vi "Update Plot.vi"(8 "error in (no error)":errorcluster, 11 "Lockin Processor in":refnum<class "Lockin Processor.lvclass">) -> (0 "error out":errorcluster, 3 "Lockin Processor out":refnum<class "Lockin Processor.lvclass">)   [LabVIEW 2015, in "Lockin Processor.lvclass"]
uses:
  Lockin Processor.lvclass
  Lockin Processor.lvclass/Lockin Processor.ctl
  Lockin Processor Configuration.ctl
  Read Lockin Processor Configuration.vi
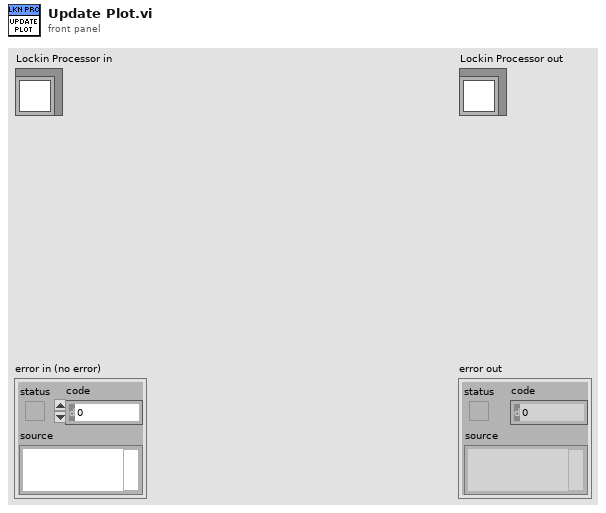
[diagram p1: front panel]
types:
  T1 = typedef "Lockin Processor Configuration.ctl" = cluster{"Time constant":dbl, "Phase":dbl, "Signal channels":string[], "Group":string, "X channel":string, "Live update":bool}
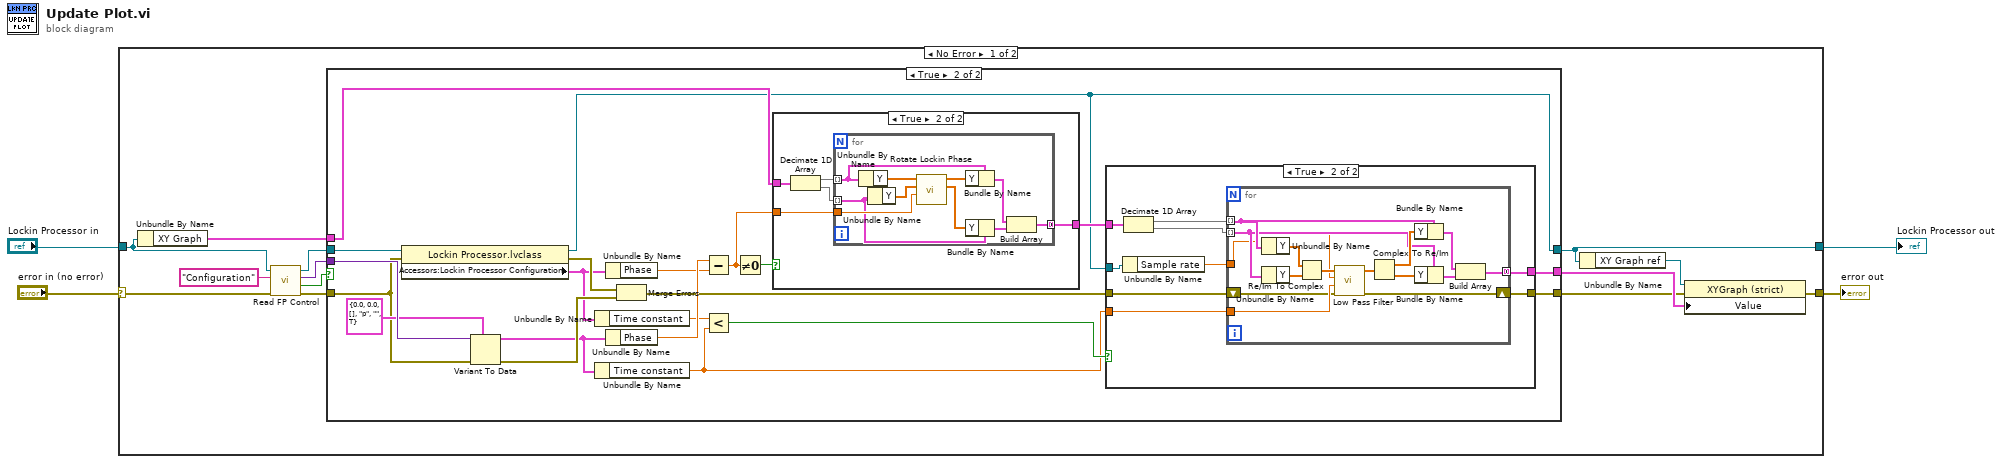
[diagram p0: block diagram]
diagram:
  n1 = case shown="No Error" "error in (no error)" {
    selector: "error in (no error)" -> [w7 w85]
    tunnel: [w6 w85] -> w3
    tunnel: [w9 w84] -> w1
    tunnel: "Lockin Processor in" -> [w10 w84]
    frame No Error {
      n2 = Unbundle By Name(w10) -> ("XY Graph"=w12:cluster{"X":dbl[], "Y":dbl[]}[])
      n3 = call-dynamic "Read FP Control.vi"("error in (no error)"=w7, "Control Name"="Configuration", "Measure Object in"=w10) -> ("error out"=w15:errorcluster, "Present"=w14:bool, "Control Value"=w16:variant, "Measure Object out"=w13:refnum<class "Lockin Processor.lvclass">)  [unwired: 5 in]
      n4 = case shown="True" w14 {
        tunnel: w16 -> [_ w41]
        tunnel: w15 -> [w18 w38]
        tunnel: w13 -> [w19 w39]
        tunnel: w12 -> [w20 w34]
        tunnel: [w19 w21] -> w9
        tunnel: [w20 w22] -> w11
        tunnel: [w18 w23] -> w5
        frame False {
        }
        frame True {
          n5 = property class="Lockin Processor.lvclass"(reference=w39, error in=w38) -> (reference out=w21:refnum<class "Lockin Processor.lvclass">, error out=w37:errorcluster, "Accessors:Lockin Processor Configuration"=w30:T1)
          n6 = Variant To Data(error in=w38, type=T1 {"Time constant"=0.0, "Phase"=0.0, "Signal channels"=[], "Group"="p", "X channel"="", "Live update"=TRUE} ("Configuration"), Variant=w41) -> (data=w29:T1, error out=w36:errorcluster)
          n7 = Unbundle By Name(w30) -> ("Time constant"=w28:dbl)
          n8 = Unbundle By Name(w29) -> ("Time constant"=w26:dbl)
          n9 = Unbundle By Name(w30) -> ("Phase"=w31:dbl)
          n10 = Unbundle By Name(w29) -> ("Phase"=w32:dbl)
          n11 = Merge Errors(w37, w36) -> (w24:errorcluster)
          n12 = Subtract(x=w32, y=w31) -> (x-y=w33:dbl)
          n13 = Less?(x=w28, y=w26) -> (x < y?=w27:bool)
          n14 = Not Equal To 0?(x=w33) -> (x != 0?=w35:bool)
          n15 = case shown="True" w35 {
            tunnel: w34 -> [w68 w73]
            tunnel: w33 -> [_ w70]
            tunnel: [w68 w69] -> w25
            frame False {
            }
            frame True {
              n16 = Decimate 1D Array(w73) -> (w72:cluster{"X":dbl[], "Y":dbl[]}[], w71:cluster{"X":dbl[], "Y":dbl[]}[])
              n17 = for {
                tunnel: w72 -> [w81] mode=indexing
                tunnel: w71 -> [w78] mode=indexing
                tunnel: w70 -> [w82]
                tunnel: [w76] -> w69 mode=concatenating
                n18 = Unbundle By Name(w81) -> ("Y"=w74:dbl[])
                n19 = Unbundle By Name(w78) -> ("Y"=w83:dbl[])
                n20 = call "Rotate Lockin Phase.vi"("Phase"=w82, "Array Y in"=w83, "Array X in"=w74) -> ("Array Y out"=w79:dbl[], "Array X out"=w80:dbl[])  [unwired: 7 in]
                n21 = Bundle By Name(cluster=w81, "Y"=w80) -> (w77:cluster{"X":dbl[], "Y":dbl[]})
                n22 = Bundle By Name(cluster=w78, "Y"=w79) -> (w75:cluster{"X":dbl[], "Y":dbl[]})
                n23 = Build Array(w77, w75) -> (w76:cluster{"X":dbl[], "Y":dbl[]}[])
              }
            }
          }
          n24 = case shown="True" w27 {
            tunnel: w25 -> [w43 w52]
            tunnel: w26 -> [_ w49]
            tunnel: [w43 w48] -> w22
            tunnel: w24 -> [w42 w47]
            tunnel: [w42 w46] -> w23
            tunnel: w21 -> [_ w45]
            frame False {
            }
            frame True {
              n25 = Unbundle By Name(w45) -> ("Sample rate"=w44:dbl)
              n26 = Decimate 1D Array(w52) -> (w51:cluster{"X":dbl[], "Y":dbl[]}[], w50:cluster{"X":dbl[], "Y":dbl[]}[])
              n27 = for {
                tunnel: w51 -> [w58] mode=indexing
                tunnel: w50 -> [w57] mode=indexing
                tunnel: w49 -> [w56]
                tunnel: [w66] -> w48 mode=concatenating
                shift-right: [w54] -> w46
                shift-left: w47 -> [w55]
                tunnel: w44 -> [w53]
                n28 = Unbundle By Name(w58) -> ("Y"=w64:dbl[])
                n29 = Unbundle By Name(w57) -> ("Y"=w63:dbl[])
                n30 = Re/Im To Complex(1:w63, 2:w64) -> (0:w62:cdb[])
                n31 = call "Low Pass Filter.vi"("Error In"=w55, "Time constant"=w56, "Sample rate"=w53, "Data"=w62) -> ("Error Out"=w54:errorcluster, "Data out"=w61:cdb[])  [unwired: 6 in]
                n32 = Complex To Re/Im(x + iy=w61) -> (x=w60:dbl[], y=w59:dbl[])
                n33 = Bundle By Name(cluster=w58, "Y"=w60) -> (w67:cluster{"X":dbl[], "Y":dbl[]})
                n34 = Bundle By Name(cluster=w57, "Y"=w59) -> (w65:cluster{"X":dbl[], "Y":dbl[]})
                n35 = Build Array(w67, w65) -> (w66:cluster{"X":dbl[], "Y":dbl[]}[])
              }
            }
          }
        }
      }
      n36 = Unbundle By Name(w9) -> ("XY Graph ref"=w8:refnum<vi>)
      n37 = property class="XYGraph (strict)"(reference=w8, error in=w5, "Value"=w11) -> (error out=w6:errorcluster)  [unwired: 1 out]
    }
    frame Error {
    }
  }
  "error out" <- w3
  "Lockin Processor out" <- w1
